vi "getColumn.vi"(8 "error in (no error)":errorcluster, 11 "object in":refnum<class "SQLiteConnection.lvclass">) -> (0 "error out":errorcluster, 2 "col text":string, 3 "object out":refnum<class "SQLiteConnection.lvclass">)   [LabVIEW 2019, in "SQLiteConnection.lvclass"]
uses:
  SQLiteConnection.lvclass
  SQLiteConnection.lvclass/SQLiteConnection.ctl
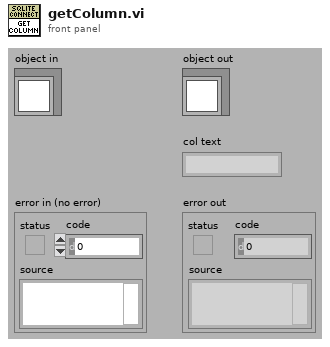
[diagram p1: front panel]
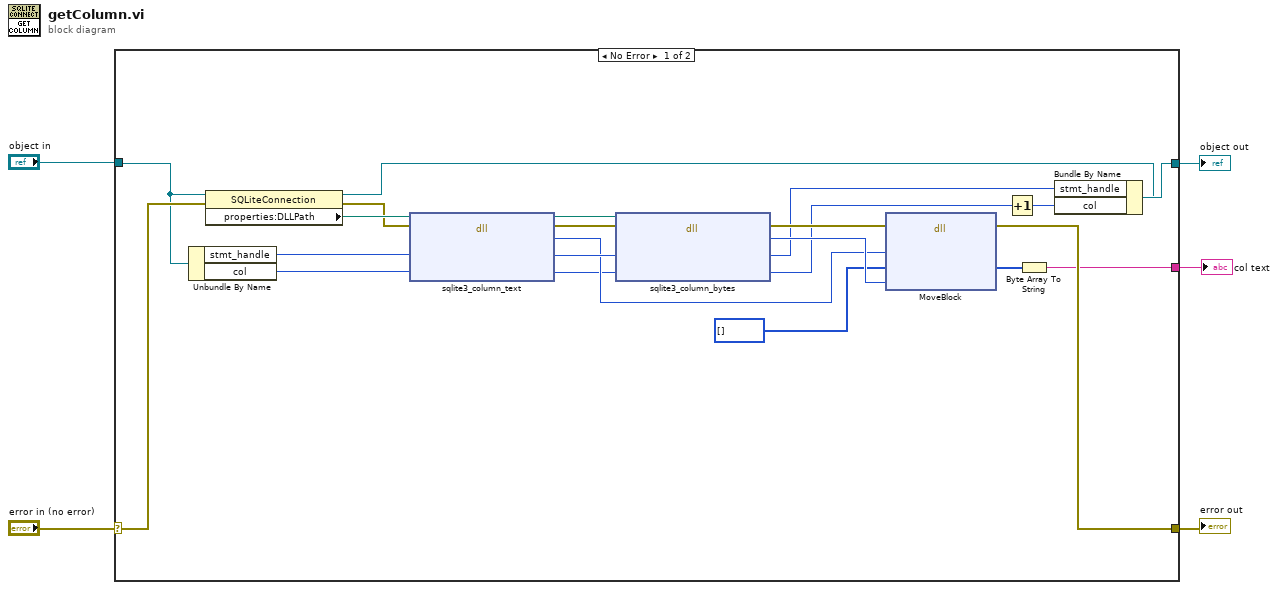
[diagram p0: block diagram]
diagram:
  n1 = case shown="No Error" "error in (no error)" {
    selector: "error in (no error)" -> [w14 w29]
    tunnel: [w7 w29] -> w4
    tunnel: [w27 w28] -> w2
    tunnel: "object in" -> [w11 w28]
    tunnel: [w6 _] -> w1
    frame No Error {
      n2 = Unbundle By Name(w11) -> ("stmt_handle"=w16:u64, "col"=w15:i32)
      n3 = property class="SQLiteConnection"(reference=w11, error in=w14) -> (reference out=w10:refnum<class "SQLiteConnection.lvclass">, error out=w12:errorcluster, "properties:DLLPath"=w13:path)
      n4 = dll-call lib="D:/Users/mcarl/Documents/LabVIEW Projects/OW-PIKO/OW-PIKO Software/sqlite3.dll" fn="sqlite3_column_text"(path in=w13, error in=w12, "stmt_pointer"=w16, "col_int"=w15) -> (path out=w23:path, error out=w22:errorcluster, "return type"=w19:u64, "stmt_pointer"=w20:u64, "col_int"=w18:i32)  [unwired: 1 in]
      n5 = dll-call lib="C:/LabVIEW_JDP/Support/SQLite/SQL Connection/sqlite3.dll" fn="sqlite3_column_bytes"(path in=w23, error in=w22, "stmt_pointer"=w20, "col_int"=w18) -> (error out=w21:errorcluster, "no bytes"=w26:i32, "stmt_pointer"=w8:u64, "col_int"=w17:i32)  [unwired: 1 in, 1 out]
      n6 = dll-call lib="LabVIEW" fn="MoveBlock"(error in=w21, "Source Pointer"=w19, "Destination U8 Array"=u8[] [], "Number of Bytes"=w26) -> (error out=w7:errorcluster, "Destination U8 Array"=w25:u8[])  [unwired: 5 in, 1 out]
      n7 = Increment(x=w17) -> (x+1=w9:i32)
      n8 = Byte Array To String(unsigned byte array=w25) -> (string=w6:string)
      n9 = Bundle By Name(cluster=w10, "stmt_handle"=w8, "col"=w9) -> (w27:refnum<class "SQLiteConnection.lvclass">)
    }
    frame Error {
    }
  }
  "error out" <- w4
  "object out" <- w2
  "col text" <- w1
